vi "SVX Buffer Shaft Centerline Plot.vi"(0 "shaft centerline in":T1(array[cluster]), 1 "buffer mode":u16(ring)=1 items=["Infinite length", "Last block data", "Custom"], 2 "reset? (F)":bool, 7 "buffer size (samples)":dbl, 11 "error in (no error)":errorcluster) -> (4 "shaft centerline out":T1(array[cluster]), 15 "error out":errorcluster)   [LabVIEW 2017, in "SoundVib_MCMDisplay.lvlib"]
doc: "Buffers shaft centerline plot data according to different buffer modes. This VI requires continuous input data. The buffered data might have gaps between or overlap with previous buffers. Do not use the buffered data for limit testing or data logging."
uses:
  <vilib>/addons/Sound and Vibration/Order Analysis/Data Presentation/SoundVib_MCMDisplay.lvlib
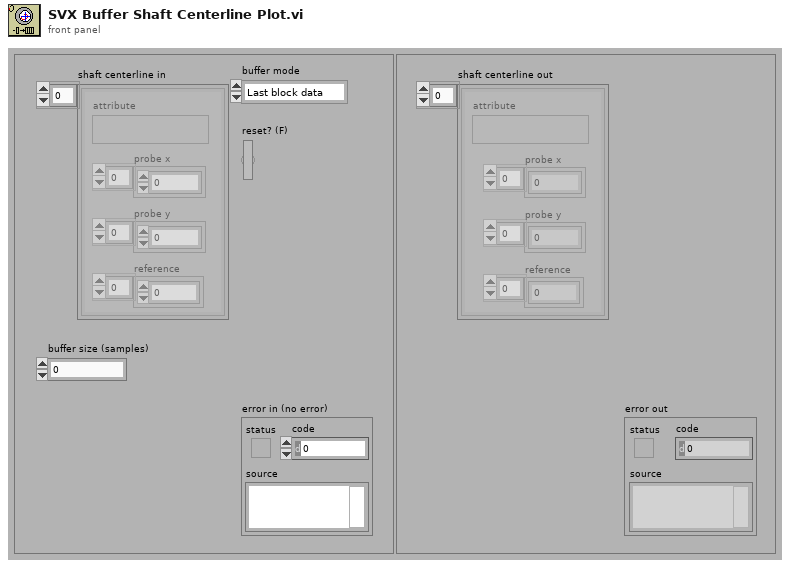
[diagram p1: front panel]
types:
  T1 = cluster{"probe x":dbl[], "probe y":dbl[], "reference":dbl[], "attribute":variant}[]
  T2 = cluster{"probe x":dbl[], "probe y":dbl[], "reference":dbl[], "attribute":variant}
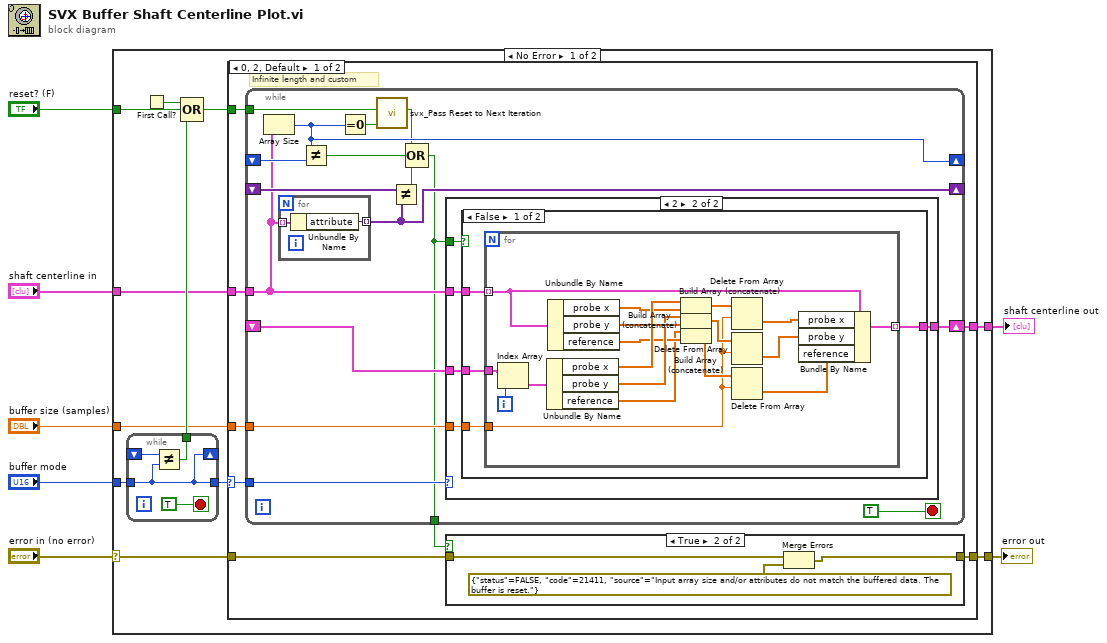
[diagram p0: block diagram]
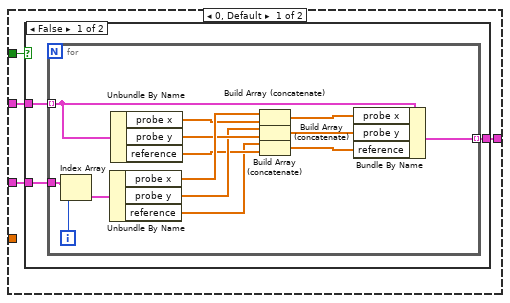
[diagram p3: hidden frame]
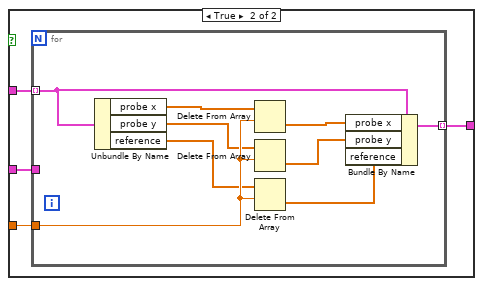
[diagram p5: hidden frame]
diagram:
  n1 = case shown="No Error" "error in (no error)" {
    selector: "error in (no error)" -> [w10 w117]
    tunnel: "buffer mode" -> [w18 _]
    tunnel: "reset? (F)" -> [w17 _]
    tunnel: "shaft centerline in" -> [w13 _]
    tunnel: "buffer size (samples)" -> [w11 _]
    tunnel: [w9 w117] -> w2
    tunnel: [w8 _] -> w1
    frame No Error {
      n2 = while {
        tunnel: w18 -> [w114]
        tunnel: [w114] -> w14
        shift-right: [w114] -> _
        shift-left: _ -> [w115]
        tunnel: [w113] -> w16
        stop <- TRUE stop-if-true
        n3 = Not Equal?(x=w115, y=w114) -> (x != y?=w113:bool)
      }
      n4 = First Call?() -> (First Call?: T/F=w15:bool)
      n5 = Compound Arithmetic op=OR(w15, w17, w16) -> (w12:bool)
      n6 = case shown="0, 2, Default" w14 {
        selector: w14 -> [w24 _]
        tunnel: w13 -> [w26 w112]
        tunnel: w12 -> [w25 _]
        tunnel: w11 -> [w23 _]
        tunnel: w10 -> [w21 w111]
        tunnel: [w20 w111] -> w9
        tunnel: [w22 w112] -> w8
        frame 0, 2, Default {
          # "Infinite length and custom"
          n7 = while {
            tunnel: w26 -> [w35]
            shift-right: [w37] -> _
            shift-left: _ -> [w38]
            shift-right: [w45] -> _
            shift-left: _ -> [w46]
            tunnel: w25 -> [w44]
            tunnel: w24 -> [w40]
            shift-right: [w34] -> w22
            shift-left: _ -> [w33]
            tunnel: w23 -> [w32]
            tunnel: [w31] -> w19
            stop <- TRUE stop-if-true
            n8 = Array Size(array=w35) -> (size(s)=w45:i32)
            n9 = for {
              tunnel: w35 -> [w110] mode=indexing
              tunnel: [w109] -> w37 mode=indexing
              n10 = Unbundle By Name(w110) -> ("attribute"=w109:variant)
            }
            n11 = Not Equal?(x=w45, y=w46) -> (x != y?=w42:bool)
            n12 = Equal To 0?(x=w45) -> (x = 0?=w43:bool)
            n13 = call <vilib>:"svx_Pass Reset to Next Iteration.vi"("trigger"=w43, "reset?(F)"=w44) -> ("reset out"=w41:bool)  [unwired: 9 in]
            n14 = Not Equal?(x=w38, y=w37) -> (x != y?=w36:bool)
            n15 = Compound Arithmetic op=OR(w41, w42, w36) -> (w31:bool)
            n16 = case shown="2" w40 {
              tunnel: w31 -> [w50 w73]
              tunnel: w35 -> [w49 w72]
              tunnel: [w48 w71] -> w34
              tunnel: w33 -> [w47 w70]
              tunnel: w32 -> [_ w69]
              frame 0, Default {
                n17 = case shown="False" w50 {
                  tunnel: w49 -> [w53 w68]
                  tunnel: [w52 w68] -> w48
                  tunnel: w47 -> [w51 _]
                  frame False {
                    n18 = for {
                      tunnel: w53 -> [w54] mode=indexing
                      tunnel: [w67] -> w52 mode=indexing
                      tunnel: w51 -> [w66]
                      i -> [w65]
                      n19 = Index Array(array=w66, index=w65) -> (element=w64:T2)
                      n20 = Unbundle By Name(w64) -> ("probe x"=w63:dbl[], "probe y"=w58:dbl[], "reference"=w55:dbl[])
                      n21 = Unbundle By Name(w54) -> ("probe x"=w62:dbl[], "probe y"=w59:dbl[], "reference"=w56:dbl[])
                      n22 = Build Array (concatenate)(w63, w62) -> (w61:dbl[])
                      n23 = Build Array (concatenate)(w58, w59) -> (w60:dbl[])
                      n24 = Build Array (concatenate)(w55, w56) -> (w57:dbl[])
                      n25 = Bundle By Name(cluster=w54, "probe x"=w61, "probe y"=w60, "reference"=w57) -> (w67:T2)
                    }
                  }
                  frame True {
                  }
                }
              }
              frame 2 {
                n26 = case shown="False" w73 {
                  tunnel: w72 -> [w77 w99]
                  tunnel: [w76 w98] -> w71
                  tunnel: w70 -> [w75 w97]
                  tunnel: w69 -> [w74 w96]
                  frame False {
                    n27 = for {
                      tunnel: w77 -> [w95] mode=indexing
                      tunnel: [w94] -> w76 mode=indexing
                      tunnel: w75 -> [w93]
                      tunnel: w74 -> [w79]
                      i -> [w92]
                      n28 = Index Array(array=w93, index=w92) -> (element=w91:T2)
                      n29 = Unbundle By Name(w91) -> ("probe x"=w90:dbl[], "probe y"=w87:dbl[], "reference"=w85:dbl[])
                      n30 = Unbundle By Name(w95) -> ("probe x"=w89:dbl[], "probe y"=w88:dbl[], "reference"=w86:dbl[])
                      n31 = Build Array (concatenate)(w90, w89) -> (w84:dbl[])
                      n32 = Build Array (concatenate)(w87, w88) -> (w83:dbl[])
                      n33 = Build Array (concatenate)(w85, w86) -> (w80:dbl[])
                      n34 = Delete From Array(array=w84, length=w79) -> (deleted portion=w82:dbl[])  [unwired: 1 in, 1 out]
                      n35 = Delete From Array(array=w83, length=w79) -> (deleted portion=w81:dbl[])  [unwired: 1 in, 1 out]
                      n36 = Delete From Array(array=w80, length=w79) -> (deleted portion=w78:dbl[])  [unwired: 1 in, 1 out]
                      n37 = Bundle By Name(cluster=w95, "probe x"=w82, "probe y"=w81, "reference"=w78) -> (w94:T2)
                    }
                  }
                  frame True {
                    n38 = for {
                      tunnel: w99 -> [w108] mode=indexing
                      tunnel: [w107] -> w98 mode=indexing
                      tunnel: w97 -> [_]
                      tunnel: w96 -> [w104]
                      n39 = Unbundle By Name(w108) -> ("probe x"=w102:dbl[], "probe y"=w101:dbl[], "reference"=w100:dbl[])
                      n40 = Delete From Array(array=w102, length=w104) -> (deleted portion=w106:dbl[])  [unwired: 1 in, 1 out]
                      n41 = Delete From Array(array=w101, length=w104) -> (deleted portion=w105:dbl[])  [unwired: 1 in, 1 out]
                      n42 = Delete From Array(array=w100, length=w104) -> (deleted portion=w103:dbl[])  [unwired: 1 in, 1 out]
                      n43 = Bundle By Name(cluster=w108, "probe x"=w106, "probe y"=w105, "reference"=w103) -> (w107:T2)
                    }
                  }
                }
              }
            }
          }
          n44 = case shown="True" w19 {
            tunnel: w21 -> [w27 w30]
            tunnel: [w27 w29] -> w20
            frame False {
            }
            frame True {
              n45 = Merge Errors(w30, errorcluster {"status"=FALSE, "code"=21411, "source"="Input array size and/or attributes do not match the buffered data. The buffer is reset."} ("error in 2 (no error)")) -> (w29:errorcluster)
            }
          }
        }
        frame 1 {
          # "Last block data"
        }
      }
    }
    frame Error {
    }
  }
  "shaft centerline out" <- w1
  "error out" <- w2
